vi "ArrayOfPicturesOut.vi"() -> (0 "Array Of Pictures":picture[](array[picture]))   [LabVIEW 2011]
panel:
  in  "picture 3":picture
  in  "picture 2":picture
  in  "picture":picture
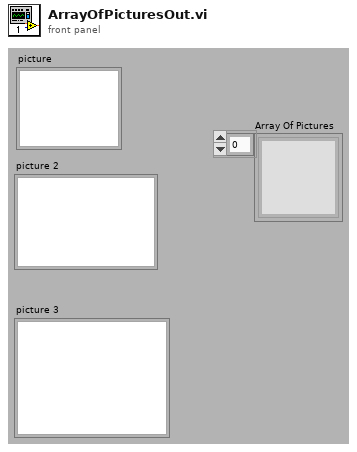
[diagram p1: front panel]
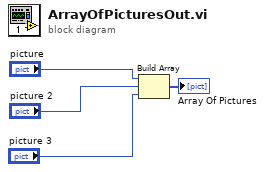
[diagram p0: block diagram]
diagram:
  n1 = Build Array("picture", "picture 2", "picture 3") -> (→"Array Of Pictures":picture[])
